vi "Initialize.vi"(8 "error in (no error)":errorcluster, 9 "Reset (T: Reset)":bool=TRUE, 10 "ID Query (T: Check)":bool=TRUE, 11 "VISA resource name":refnum<visa-resource-name>) -> (0 "error out":errorcluster, 3 "VISA resource name out":refnum<visa-resource-name>)   [LabVIEW 2020, in "Rohde&Schwarz CMXP NR FR2 Measurement.lvlib"]
doc: "This VI open a new connection to the instrument.\nOptionally, you can reset the instrument.\nSetting *IDN? query to False will skip checking of the supported driver's instrument types.\nYou must run this VI or <b>Initialize with Options.vi</b> before using any of the instrument driver VIs."
uses:
  <instrlib>/Rohde&Schwarz CMXP NR FR2 Measurement/Rohde&Schwarz CMXP NR FR2 Measurement.lvlib
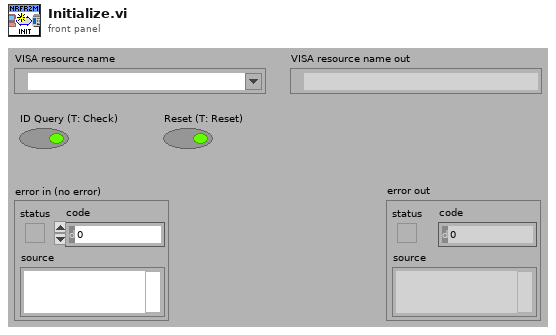
[diagram p1: front panel]
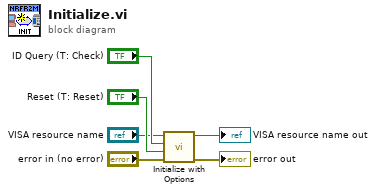
[diagram p0: block diagram]
diagram:
  n1 = call <instrlib>:"Initialize with Options.vi"("error in (no error)"="error in (no error)", "Reset (T: Reset)"="Reset (T: Reset)", "ID Query (T: Check)"="ID Query (T: Check)", "VISA resource name"="VISA resource name") -> ("error out"=→"error out":errorcluster, "VISA resource name out"=→"VISA resource name out":refnum<visa-resource-name>)  [unwired: 6 in]
